vi "PH_gentec_Powermeter.ProcCases.vi"(0 "i ref in":refnum<vi>, 1 "selector":string, 2 "Data":T1, 3 "call cluster":T2={"Object"="", "Selector"="", "CallType"=enum."synchronous", "Async Object"="", "Async Selector"="", "Data Descriptor"="", "Data"=[], "Error #"=0, "Expire"=0}, 5 "error in":errorcluster) -> (14 "i ref out":refnum<vi>, 17 "answer cluster":T2={"Object"="", "Selector"="", "CallType"=enum."synchronous", "Async Object"="", "Async Selector"="", "Data Descriptor"="", "Data"=[], "Error #"=0, "Expire"=0}, 19 "error out":errorcluster)   [LabVIEW 2014, in "PH_gentec_Powermeter.lvlib"]
doc: "This method is called by a process from within the default case in the event loop. The methods of a class that are linked to events will be called from THIS method. Add your code here."
uses:
  PH_gentec_Powermeter.lvlib
  CSCore/CSSystem/CoreDefs/CoreDefs.call_type.ctl
  CSCore/BaseProcess/BaseProcess.descriptor string definition.ctl
  CSCore/CSSystem/CoreDefs/CoreDefs.rawDataType.ctl
  non_GPL/instr.lib/gentec-SOLO-PE/Driver/Type Defs/gentec-SOLO-PE.Data Sampling Settings.ctl
  CSCore/CSSystem/CoreLib/CoreLib.byte array 2 short.vi
  CSCore/CSSystem/CoreLib/CoreLib.string 2 byte array.vi
  CSCore/CSSystem/CoreLib/CoreLib.byte array 2 int.vi
  CSCore/CSSystem/CoreLib/CoreLib.lvlib
  CSCore/BaseProcess/BaseProcess.lvlib
  CSCore/CAEObj/CAEObj.lvlib
  PH_PSDBWriter/PH_PSDBWriter.lvlib
  PH_Powermeter_BaseClass/PH_Powermeter_BaseClass.lvlib
  non_GPL/instr.lib/gentec-SOLO-PE/gentec-SOLO-PE - Driver.lvlib
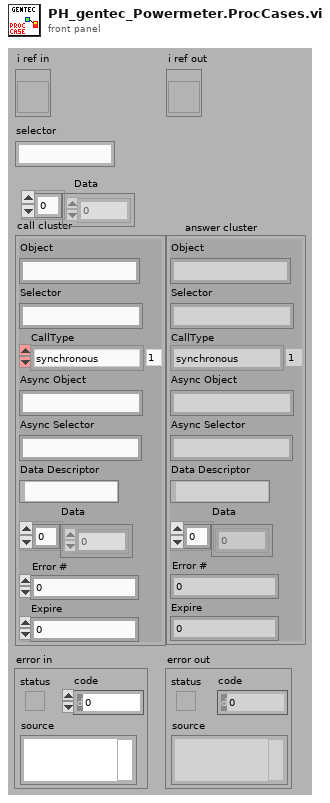
[diagram p1: front panel]
types:
  T1 = typedef "CoreDefs.rawDataType.ctl" = i8[]
  T2 = typedef "CoreDefs.call_type.ctl" = cluster{"Object":string, "Selector":string, "CallType":enum16{"simple", "synchronous", "asynchronous"}, "Async Object":string, "Async Selector":string, "Data Descriptor":T3, "Data":T1, "Error #":i32, "Expire":u32}
  T3 = typedef "BaseProcess.lvlib/BaseProcess.descriptor string definition.ctl" = string
  T4 = typedef "gentec-SOLO-PE - Driver.lvlib/gentec-SOLO-PE.Data Sampling Settings.ctl" = cluster{"Sample Rate":u32, "Sample Rate Unit":u32, "Sample Period":u32, "Sample Period Unit":u32, "Total Duration":u32, "Total Duration Unit":u32, "Time Stamp":u32}
  T5 = typedef "PH_PSDBWriter.lvlib/PH_PSDBWriter.PHELIX-Subsystems.ctl" = i32
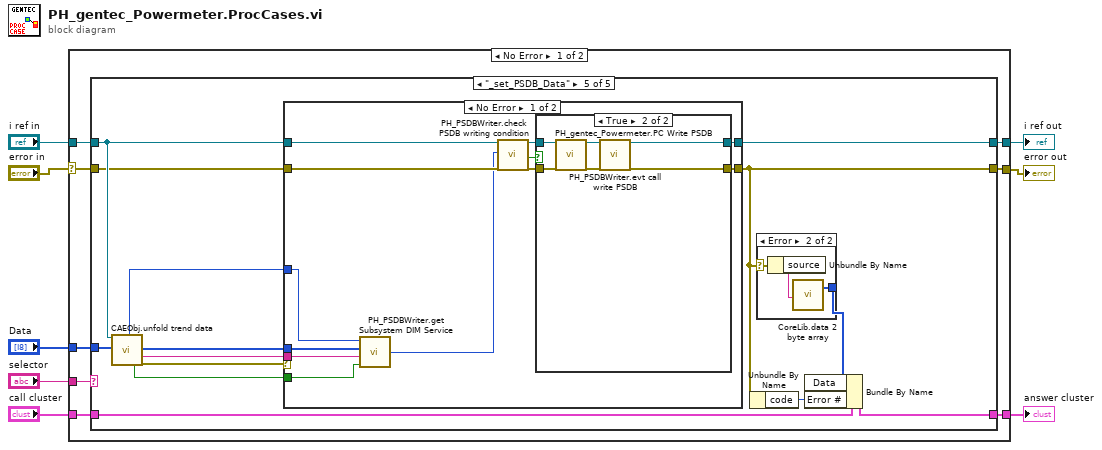
[diagram p0: block diagram]
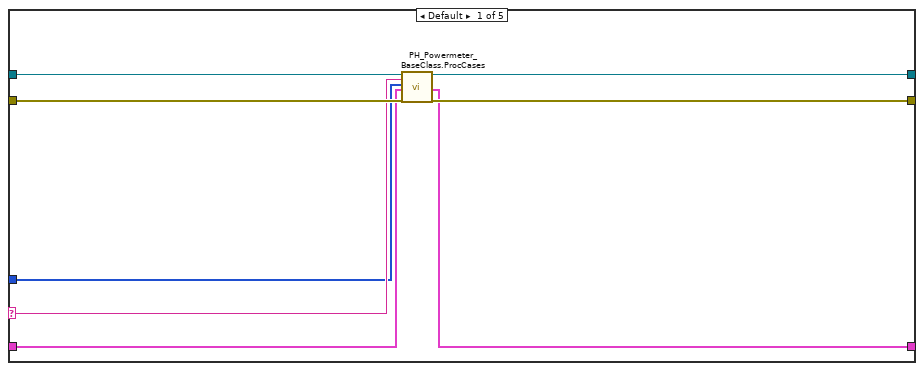
[diagram p2: hidden frame]
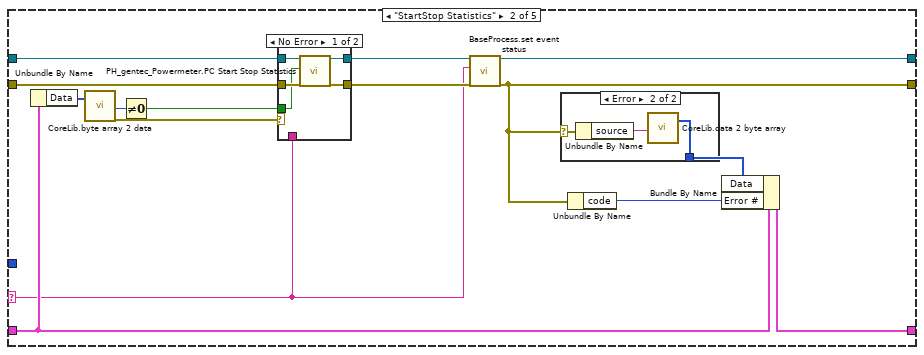
[diagram p3: hidden frame]
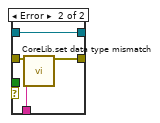
[diagram p5: hidden frame]
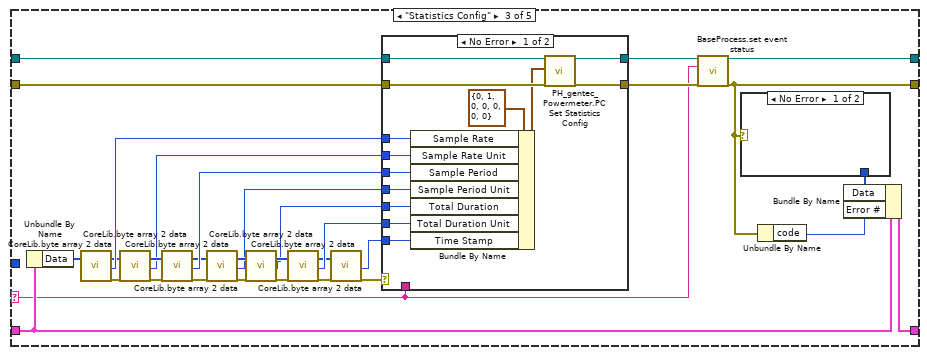
[diagram p6: hidden frame]
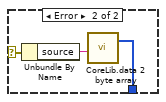
[diagram p7: hidden frame]
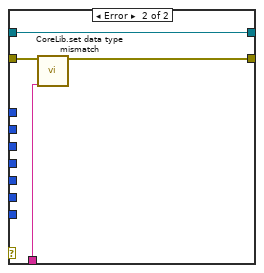
[diagram p8: hidden frame]
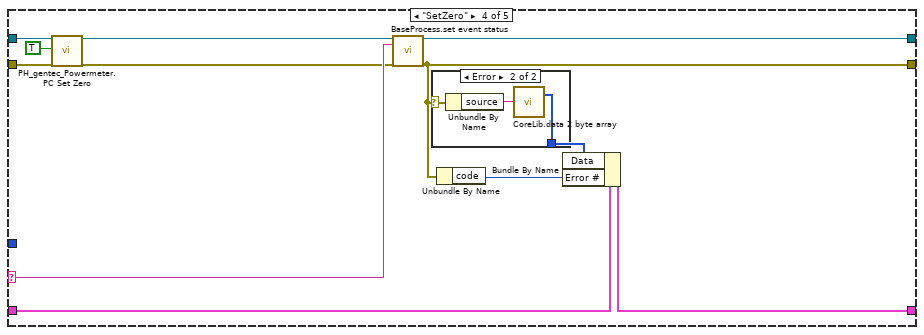
[diagram p9: hidden frame]
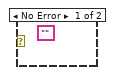
[diagram p10: hidden frame]
diagram:
  n1 = case shown="No Error" "error in" {
    selector: "error in" -> [w9 w159]
    tunnel: "selector" -> [w16 _]
    tunnel: [w15 w158] -> w7
    tunnel: "call cluster" -> [w14 w158]
    tunnel: "i ref in" -> [w13 w160]
    tunnel: [w12 w160] -> w4
    tunnel: [w11 w159] -> w1
    tunnel: "Data" -> [w10 _]
    frame No Error {
      n2 = case shown="\"_set_PSDB_Data\"" w16 {
        selector: w16 -> [w19 w31 w77 w111 _]
        tunnel: w13 -> [w18 w39 w83 w107 w123]
        tunnel: [w24 w32 w76 w112 w122] -> w12
        tunnel: w14 -> [w20 w36 w80 w114 w131]
        tunnel: [w21 w35 w72 w109 w129] -> w15
        tunnel: w9 -> [w23 w38 w82 w108 w120]
        tunnel: [w22 w33 w75 w113 w121] -> w11
        tunnel: w10 -> [w17 _ _ _ w119]
        frame Default {
          # "In the default case, always call the ProcCase method of the parent class"
          n3 = call "PH_Powermeter_BaseClass.ProcCases.vi"("i ref in"=w18, "selector"=w19, "Data"=w17, "call cluster"=w20, "error in"=w23) -> ("i ref out"=w24:refnum<vi>, "answer cluster"=w21:T2, "error out"=w22:errorcluster)  [unwired: 12 in]
        }
        frame "StartStop Statistics" {
          n4 = Unbundle By Name(w36) -> ("Data"=w27:T1)
          n5 = call-poly "CoreLib.byte array 2 data.vi"("byteArray"=w27) -> ("i16"=w29:i16, "error out"=w26:errorcluster)  [unwired: 16 in, 1 out]
          n6 = Not Equal To 0?(x=w29) -> (x != 0?=w28:bool)
          n7 = case shown="No Error" w26 {
            tunnel: [w44 w51] -> w30
            tunnel: w39 -> [w47 w51]
            tunnel: w38 -> [w46 w50]
            tunnel: [w43 w49] -> w34
            tunnel: w31 -> [_ w48]
            tunnel: w28 -> [w45 _]
            frame No Error {
              n8 = call "PH_gentec_Powermeter.PC Start Stop Statistics.vi"("VI in"=w47, "Start / Stop Statistics"=w45, "error in (no error)"=w46) -> ("VI out"=w44:refnum<vi>, "error out"=w43:errorcluster)  [unwired: 15 in]
            }
            frame Error {
              n9 = call "CoreLib.set data type mismatch.vi"("error in (no error)"=w50, "error source"=w48) -> ("error out"=w49:errorcluster)  [unwired: 17 in]
            }
          }
          n10 = call "BaseProcess.set event status.vi"("i ref in"=w30, "EventStatus"=w31, "error in (no error)"=w34) -> ("i ref out"=w32:refnum<vi>, "error out"=w33:errorcluster)  [unwired: 14 in, 1 out]
          n11 = case shown="Error" w33 {
            selector: w33 -> [_ w42]
            tunnel: [_ w40] -> w25
            frame No Error {
            }
            frame Error {
              n12 = Unbundle By Name(w42) -> ("source"=w41:string)
              n13 = call-poly "CoreLib.data 2 byte array.vi"("string"=w41) -> ("byteArray out"=w40:T1)  [unwired: 18 in]
            }
          }
          n14 = Unbundle By Name(w33) -> ("code"=w37:i32)
          n15 = Bundle By Name(cluster=w36, "Data"=w25, "Error #"=w37) -> (w35:T2)
        }
        frame "Statistics Config" {
          n16 = Unbundle By Name(w80) -> ("Data"=w74:T1)
          n17 = call-poly "CoreLib.byte array 2 data.vi"("byteArray"=w74) -> ("byteArray out"=w68:T1, "i32"=w73:i32, "error out"=w70:errorcluster)  [unwired: 16 in]
          n18 = call-poly "CoreLib.byte array 2 data.vi"("byteArray"=w68, "error in (no error)"=w70) -> ("byteArray out"=w67:T1, "i32"=w66:i32, "error out"=w69:errorcluster)  [unwired: 15 in]
          n19 = call-poly "CoreLib.byte array 2 data.vi"("byteArray"=w67, "error in (no error)"=w69) -> ("byteArray out"=w57:T1, "i32"=w65:i32, "error out"=w60:errorcluster)  [unwired: 15 in]
          n20 = call-poly "CoreLib.byte array 2 data.vi"("byteArray"=w57, "error in (no error)"=w60) -> ("byteArray out"=w62:T1, "i32"=w56:i32, "error out"=w64:errorcluster)  [unwired: 15 in]
          n21 = call-poly "CoreLib.byte array 2 data.vi"("byteArray"=w62, "error in (no error)"=w64) -> ("byteArray out"=w61:T1, "i32"=w55:i32, "error out"=w63:errorcluster)  [unwired: 15 in]
          n22 = call-poly "CoreLib.byte array 2 data.vi"("byteArray"=w61, "error in (no error)"=w63) -> ("byteArray out"=w53:T1, "i32"=w54:i32, "error out"=w59:errorcluster)  [unwired: 15 in]
          n23 = call-poly "CoreLib.byte array 2 data.vi"("byteArray"=w53, "error in (no error)"=w59) -> ("i32"=w52:i32, "error out"=w58:errorcluster)  [unwired: 15 in, 1 out]
          n24 = case shown="No Error" w58 {
            tunnel: [w88 w103] -> w79
            tunnel: w83 -> [w99 w103]
            tunnel: w82 -> [w98 w102]
            tunnel: [w87 w101] -> w78
            tunnel: w77 -> [_ w100]
            tunnel: w73 -> [w94 _]
            tunnel: w66 -> [w95 _]
            tunnel: w65 -> [w96 _]
            tunnel: w56 -> [w92 _]
            tunnel: w55 -> [w91 _]
            tunnel: w54 -> [w90 _]
            tunnel: w52 -> [w89 _]
            frame No Error {
              n25 = Bundle By Name(cluster=T4 {"Sample Rate"=0, "Sample Rate Unit"=1, "Sample Period"=0, "Sample Period Unit"=0, "Total Duration"=0, "Total Duration Unit"=0, "Time Stamp"=0} ("Data Sampling Settings"), "Sample Rate"=w94, "Sample Rate Unit"=w95, "Sample Period"=w96, "Sample Period Unit"=w92, "Total Duration"=w91, "Total Duration Unit"=w90, "Time Stamp"=w89) -> (w93:T4)
              n26 = call "PH_gentec_Powermeter.PC Set Statistics Config.vi"("VI in"=w99, "Data Sampling Settings"=w93, "error in (no error)"=w98) -> ("VI out"=w88:refnum<vi>, "error out"=w87:errorcluster)  [unwired: 15 in]
            }
            frame Error {
              n27 = call "CoreLib.set data type mismatch.vi"("error in (no error)"=w102, "error source"=w100) -> ("error out"=w101:errorcluster)  [unwired: 17 in]
            }
          }
          n28 = call "BaseProcess.set event status.vi"("i ref in"=w79, "EventStatus"=w77, "error in (no error)"=w78) -> ("i ref out"=w76:refnum<vi>, "error out"=w75:errorcluster)  [unwired: 14 in, 1 out]
          n29 = case shown="No Error" w75 {
            selector: w75 -> [_ w86]
            tunnel: [_ w84] -> w71
            frame No Error {
            }
            frame Error {
              n30 = Unbundle By Name(w86) -> ("source"=w85:string)
              n31 = call-poly "CoreLib.data 2 byte array.vi"("string"=w85) -> ("byteArray out"=w84:T1)  [unwired: 18 in]
            }
          }
          n32 = Unbundle By Name(w75) -> ("code"=w81:i32)
          n33 = Bundle By Name(cluster=w80, "Data"=w71, "Error #"=w81) -> (w72:T2)
        }
        frame "SetZero" {
          n34 = call "PH_gentec_Powermeter.PC Set Zero.vi"("VI in"=w107, "Set Zero"=TRUE, "error in (no error)"=w108) -> ("VI out"=w105:refnum<vi>, "error out"=w104:errorcluster)  [unwired: 15 in]
          n35 = call "BaseProcess.set event status.vi"("i ref in"=w105, "EventStatus"=w111, "error in (no error)"=w104) -> ("i ref out"=w112:refnum<vi>, "error out"=w113:errorcluster)  [unwired: 14 in, 1 out]
          n36 = case shown="Error" w113 {
            selector: w113 -> [_ w118]
            tunnel: [_ w116] -> w110
            frame No Error {
              (unwired) ""
            }
            frame Error {
              n37 = Unbundle By Name(w118) -> ("source"=w117:string)
              n38 = call-poly "CoreLib.data 2 byte array.vi"("string"=w117) -> ("byteArray out"=w116:T1)  [unwired: 18 in]
            }
          }
          n39 = Unbundle By Name(w113) -> ("code"=w115:i32)
          n40 = Bundle By Name(cluster=w114, "Data"=w110, "Error #"=w115) -> (w109:T2)
        }
        frame "_set_PSDB_Data" {
          n41 = call "CAEObj.unfold trend data.vi"("i ref in"=w123, "raw trend data"=w119) -> ("quality"=w128:i32, "no link"=w125:bool, "data"=w127:i8[], "typeDescriptor"=w126:string, "error out"=w124:errorcluster)  [unwired: 9 in, 4 out]
          n42 = case shown="No Error" w124 {
            tunnel: w120 -> [w144 w154]
            tunnel: [w143 w153] -> w122
            tunnel: [w142 w154] -> w121
            tunnel: w123 -> [w140 w153]
            tunnel: w125 -> [w134 _]
            tunnel: w126 -> [w135 _]
            tunnel: w127 -> [w136 _]
            tunnel: w128 -> [w133 _]
            frame No Error {
              n43 = call "PH_PSDBWriter.get Subsystem DIM Service.vi"("no link"=w134, "typeDescriptor"=w135, "data"=w136, "quality"=w133) -> ("PHELIX Subsystems"=w137:T5)
              n44 = call "PH_PSDBWriter.check PSDB writing condition.vi"("i ref in"=w140, "wanted Subsystem"=w137, "error IO"=w144) -> ("i ref out"=w139:refnum<vi>, "write PSDB?"=w138:bool, "error out"=w141:errorcluster)  [unwired: 14 in]
              n45 = case shown="True" w138 {
                tunnel: w141 -> [w145 w152]
                tunnel: [w146 w149] -> w143
                tunnel: [w145 w147] -> w142
                tunnel: w139 -> [w146 w151]
                frame False {
                }
                frame True {
                  n46 = call "PH_gentec_Powermeter.PC Write PSDB.vi"("i ref in"=w151, "error IO"=w152) -> ("i ref out"=w150:refnum<vi>, "error out"=w148:errorcluster)  [unwired: 16 in]
                  n47 = call "PH_PSDBWriter.evt call write PSDB.vi"("i ref in"=w150, "error in (no error)"=w148) -> ("i ref out"=w149:refnum<vi>, "error out"=w147:errorcluster)  [unwired: 16 in]
                }
              }
            }
            frame Error {
            }
          }
          n48 = Unbundle By Name(w121) -> ("code"=w132:i32)
          n49 = case shown="Error" w121 {
            selector: w121 -> [_ w157]
            tunnel: [_ w155] -> w130
            frame No Error {
              (unwired) ""
            }
            frame Error {
              n50 = Unbundle By Name(w157) -> ("source"=w156:string)
              n51 = call-poly "CoreLib.data 2 byte array.vi"("string"=w156) -> ("byteArray out"=w155:T1)  [unwired: 18 in]
            }
          }
          n52 = Bundle By Name(cluster=w131, "Data"=w130, "Error #"=w132) -> (w129:T2)
        }
      }
    }
    frame Error {
    }
  }
  "answer cluster" <- w7
  "i ref out" <- w4
  "error out" <- w1
